vi "dZj(r,theta).vi"(4 "error in (no error)":errorcluster, 5 "theta":dbl, 6 "r":dbl, 7 "j (1)":i32=1) -> (0 "error out":errorcluster, 3 "dZj(r,theta)":T1)   [LabVIEW 2020, in "Zernike Polynome.lvlib"]
doc: "This VI calculates the derivative of Zj(r,theta) in x- and y-directions."
uses:
  Zernike Polynome.lvlib
  dZj(r,theta).ctl
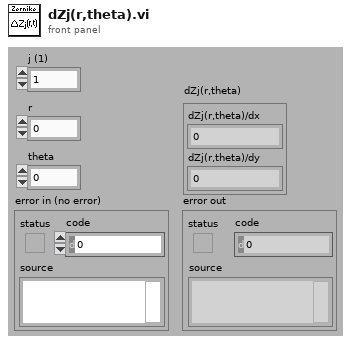
[diagram p1: front panel]
types:
  T1 = typedef "Zernike Polynome.lvlib/dZj(r,theta).ctl" = cluster{"dZj(r,theta)/dx":dbl, "dZj(r,theta)/dy":dbl}
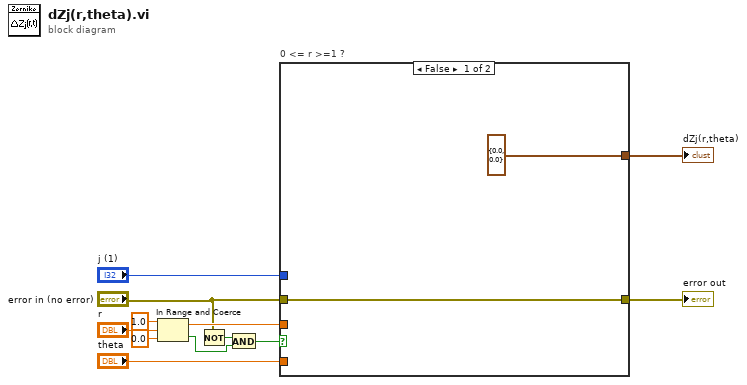
[diagram p0: block diagram]
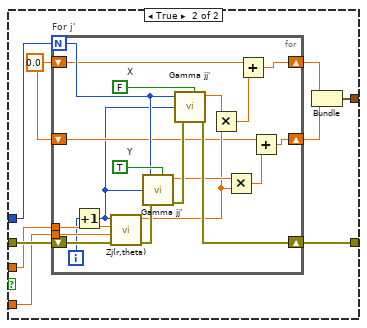
[diagram p2: hidden frame]
diagram:
  n1 = In Range and Coerce(upper limit=1.0, x="r", lower limit=0.0) -> (coerced(x)=w9:dbl, In Range?=w1:bool)
  n2 = Not(x="error in (no error)") -> (.not. x?=w2:bool)
  n3 = And(x=w2, y=w1) -> (x .and. y?=w4:bool)
  n4 = case "0 <= r >=1 ?" shown="False" w4 {
    tunnel: "error in (no error)" -> [w14 w23]
    tunnel: [cluster{dbl, dbl} {0.0, 0.0} w15] -> w5
    tunnel: "j (1)" -> [_ w19]
    tunnel: "theta" -> [_ w20]
    tunnel: w9 -> [_ w21]
    tunnel: [w14 w22] -> w6
    frame False {
    }
    frame True {
      w18 = 0.0
      n5 = for "For j'" {
        N: w19 -> [w33]
        tunnel: w21 -> [w42]
        tunnel: w20 -> [w41]
        shift-right: [w35] -> w22
        shift-left: w23 -> [w43]
        shift-right: [w29] -> w17
        shift-left: w18 -> [w28]
        shift-right: [w26] -> w16
        shift-left: w18 -> [w25]
        i -> [w40]
        w37 = TRUE  # Y
        w38 = FALSE  # X
        n6 = Increment(x=w40) -> (x+1=w24:i32)
        n7 = call "Zj(r,theta).vi"("error in (no error)"=w43, "theta"=w41, "r"=w42, "j (1)"=w24) -> ("error out"=w36:errorcluster, "Zj(r,theta)"=w31:dbl)  [unwired: 2 out]
        n8 = call "Gamma jj'.vi"("X/Y"=w37, "error in (no error)"=w36, "j' (1)"=w24, "j (1)"=w33) -> ("error out"=w39:errorcluster, "Gamma Magnitude"=w32:dbl)  [unwired: 2 out]
        n9 = call "Gamma jj'.vi"("X/Y"=w38, "error in (no error)"=w39, "j' (1)"=w24, "j (1)"=w33) -> ("error out"=w35:errorcluster, "Gamma Magnitude"=w34:dbl)  [unwired: 2 out]
        n10 = Multiply(x=w34, y=w31) -> (x*y=w30:dbl)
        n11 = Multiply(x=w32, y=w31) -> (x*y=w27:dbl)
        n12 = Add(x=w28, y=w30) -> (x+y=w29:dbl)
        n13 = Add(x=w25, y=w27) -> (x+y=w26:dbl)
      }
      n14 = Bundle(w17, w16) -> (w15:cluster{dbl, dbl})  [unwired: 1 in]
    }
  }
  "error out" <- w6
  "dZj(r,theta)" <- w5
